vi "RSZVB Select Ratios.vi"(7 "Ratios (0: b2/a1 Src Port 1)":i32(ring) items=["b2/a1 Src Port 1", "b1/a1 Src Port 1", "b2/b1 Src Port 1", "b1/b2 Src Port 1"], 8 "error in (no error)":errorcluster {"code" format="%.0x"}, 9 "Trace Name (Trc1)":string="Trc1", 10 "Channel (1)":i32=1, 11 "VISA session":refnum<visa-resource-name>) -> (0 "error out":errorcluster {"code" format="%.0x"}, 3 "dup VISA session":refnum<visa-resource-name>)   [LabVIEW 2011]
doc: "This VI select predefined complex ratios of the standard 2-port wave quantities a1, a2, b1, and b2.\n\nAssigns a measurement parameter to an existing trace or creates a trace and assigns a channel number, a name and a measurement parameter to it. The trace is not displayed.\n\nThe predefined wave quantities are all obtained with the same test set configuration, port 1 providing the stimulus signal (source port 1, forward measurement if the stimulus signal is fed to the input of the DUT). \n\nRemote-control command(s):\nCALCulate<Ch>:PARameter:SDEFine '<string>', 'B2D1/A1D1' | 'B1D1/A1D1' | 'B2D1/B1D1' | 'B1D1/B2D1'\nCALCulate<Ch>:PARameter:MEASure '<string>', 'B2D1/A1D1' | 'B1D1/A1D1' | 'B2D1/B1D1' | 'B1D1/B2D1'"
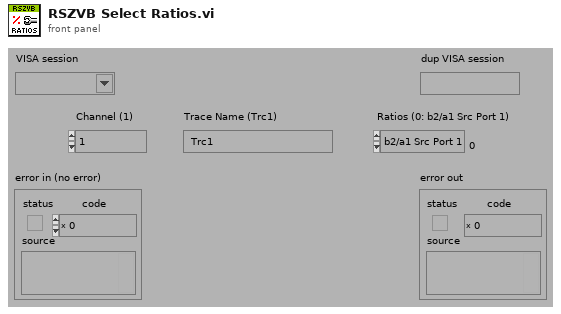
[diagram p1: front panel]
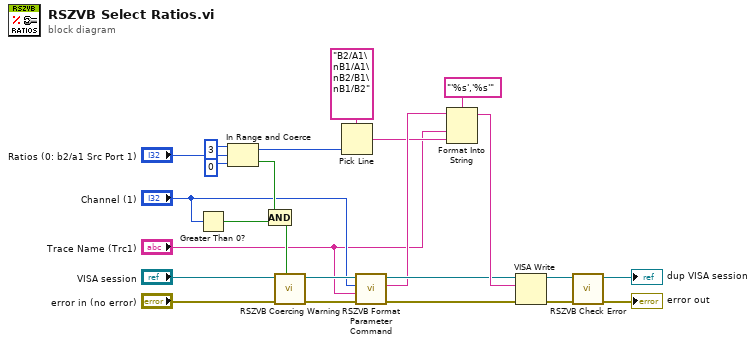
[diagram p0: block diagram]
diagram:
  n1 = Greater Than 0?(x="Channel (1)") -> (x > 0?=w9:bool)
  n2 = In Range and Coerce(upper limit=3, x="Ratios (0: b2/a1 Src Port 1)", lower limit=0) -> (coerced(x)=w12:i32, In Range?=w10:bool)
  n3 = Compound Arithmetic op=AND(w10, w9) -> (w21:bool)
  n4 = call "RSZVB Coercing Warning.vi"("In Range?"=w21, "error in (no error)"="error in (no error)", "VISA session"="VISA session") -> ("error out"=w18:errorcluster, "dup VISA session"=w17:refnum<visa-resource-name>)  [unwired: 7 in]
  n5 = Pick Line(multi-line string="B2/A1\nB1/A1\nB2/B1\nB1/B2", line index=w12) -> (output string=w11:string)  [unwired: 1 in]
  n6 = call "RSZVB Format Parameter Command.vi"("error in (no error)"=w18, "Trace Name (Trc1)"="Trace Name (Trc1)", "Channel (1)"="Channel (1)", "VISA session"=w17) -> ("error out"=w19:errorcluster, "Buffer"=w15:string, "dup VISA session"=w16:refnum<visa-resource-name>)  [unwired: 5 in]
  n7 = Format Into String(format string="'%s','%s'", initial string=w15, "Trace Name (Trc1)", w11) -> (resulting string=w20:string)  [unwired: 1 in, 1 out]
  n8 = VISA Write(VISA resource name=w16, write buffer=w20, error in (no error)=w19) -> (VISA resource name out=w22:refnum<visa-resource-name>, error out=w23:errorcluster)  [unwired: 1 out]
  n9 = call "RSZVB Check Error.vi"("error in (no error)"=w23, "VISA session"=w22) -> ("error out"=→"error out":errorcluster, "dup VISA session"=→"dup VISA session":refnum<visa-resource-name>)  [unwired: 8 in]
